vi "TryGetGraphVizPath.vi"() -> (2 "Found?":bool, 3 "Path":string)   [LabVIEW 2014]
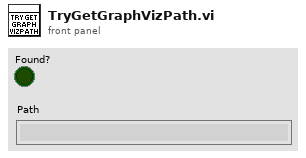
[diagram p1: front panel]
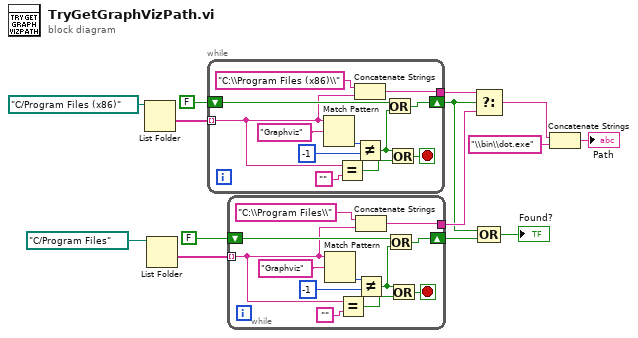
[diagram p0: block diagram]
diagram:
  n1 = List Folder(path=path "C:/Program Files (x86)") -> (folder names=w8:string[])  [unwired: 3 in, 3 out]
  n2 = List Folder(path=path "C:/Program Files") -> (folder names=w12:string[])  [unwired: 3 in, 3 out]
  n3 = while {
    tunnel: w8 -> [w19] mode=indexing
    shift-right: [w24] -> w5
    shift-left: FALSE -> [w25]
    tunnel: [w20] -> w6
    stop <- w15 stop-if-true
    n4 = Match Pattern(string=w19, regular expression="Graphviz") -> (offset past match=w23:i32)  [unwired: 1 in, 3 out]
    n5 = Equal?(x=w19, y="") -> (x = y?=w16:bool)
    n6 = Concatenate Strings("C:\\Program Files (x86)\\", w19) -> (w20:string)
    n7 = Not Equal?(x=w23, y=-1) -> (x != y?=w17:bool)
    n8 = Or(x=w25, y=w17) -> (x .or. y?=w24:bool)
    n9 = Or(x=w17, y=w16) -> (x .or. y?=w15:bool)
  }
  n10 = while {
    tunnel: w12 -> [w31] mode=indexing
    shift-right: [w36] -> w10
    shift-left: FALSE -> [w37]
    tunnel: [w32] -> w11
    stop <- w27 stop-if-true
    n11 = Match Pattern(string=w31, regular expression="Graphviz") -> (offset past match=w35:i32)  [unwired: 1 in, 3 out]
    n12 = Equal?(x=w31, y="") -> (x = y?=w28:bool)
    n13 = Concatenate Strings("C:\\Program Files\\", w31) -> (w32:string)
    n14 = Not Equal?(x=w35, y=-1) -> (x != y?=w29:bool)
    n15 = Or(x=w37, y=w29) -> (x .or. y?=w36:bool)
    n16 = Or(x=w29, y=w28) -> (x .or. y?=w27:bool)
  }
  n17 = Select(t=w6, s=w5, f=w11) -> (s? t:f=w4:string)
  n18 = Compound Arithmetic op=OR(w5, w10) -> (→"Found?":bool)
  n19 = Concatenate Strings(w4, "\\bin\\dot.exe" ("string")) -> (→"Path":string)
